vi "Run.vi"(8 "error in (no error)":errorcluster, 11 "GVIWebProcessorApp in":refnum<class "GVIWebProcessorApp.lvclass">) -> (0 "error out":errorcluster, 3 "GVIWebProcessorApp out":refnum<class "GVIWebProcessorApp.lvclass">)   [LabVIEW 2020, in "PicoG-Processor.lvlib" / "GVIWebProcessorApp.lvclass"]
uses:
  GVIWebProcessorApp.lvclass
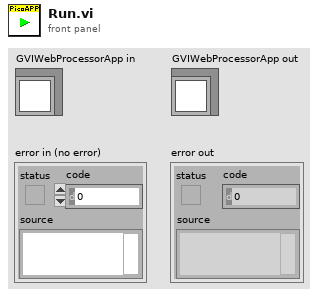
[diagram p1: front panel]
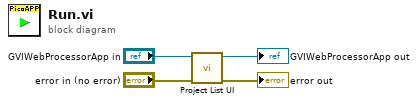
[diagram p0: block diagram]
diagram:
  n1 = call "Project List UI.vi"("error in (no error)"="error in (no error)", "GVIWebProcessorApp in"="GVIWebProcessorApp in") -> ("error out"=→"error out":errorcluster, "GVIWebProcessorApp out"=→"GVIWebProcessorApp out":refnum<class "GVIWebProcessorApp.lvclass">)  [unwired: 8 in]
